vi "Write I32.vi"(10 "I32":i32, 11 "Event in":refnum<class "Event I32.lvclass">) -> (3 "Event out":refnum<class "Event I32.lvclass">)   [LabVIEW 2016, in "Event Source.lvlib" / "Event I32.lvclass"]
uses:
  Event I32.lvclass
  Event I32.lvclass/Event I32.ctl
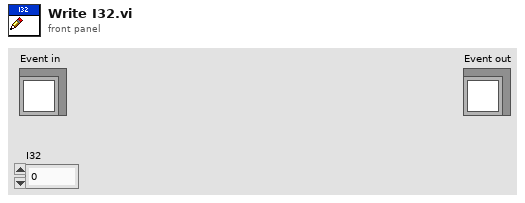
[diagram p1: front panel]
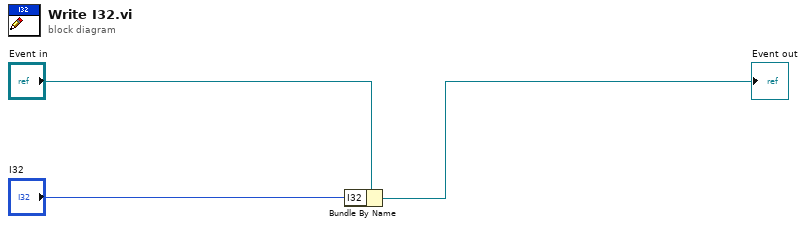
[diagram p0: block diagram]
diagram:
  n1 = Bundle By Name(cluster="Event in", "I32"="I32") -> (→"Event out":refnum<class "Event I32.lvclass">)
